vi "Display Hardware Devices.vi"(8 "error in (no error)":errorcluster, 9 "Hardware Type":string, 10 "Array of Hardware Device Names":string[](array[string]), 11 "Operator UI in":refnum<class "Measurement UI.lvclass">) -> (0 "error out":errorcluster, 3 "Operator UI out":refnum<class "Measurement UI.lvclass">)   [LabVIEW 2017, in "Measurement UI.lvlib" / "Measurement UI.lvclass"]
uses:
  Measurement UI.lvclass
  Measurement UI.lvclass/Measurement UI.ctl
  Read Multimeter.vi
  Accessors/Read Digitizer.vi
  Accessors/Read Function Generator.vi
  Accessors/Read Power Supply.vi
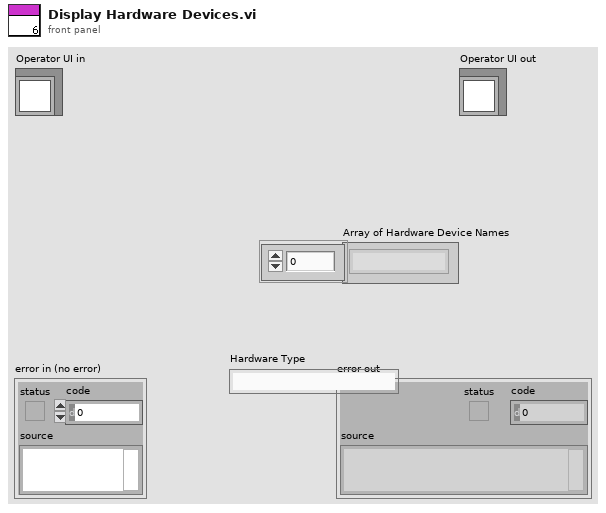
[diagram p1: front panel]
types:
  T1 = enum8{"Enabled", "Disabled", "Disabled and Grayed Out"}
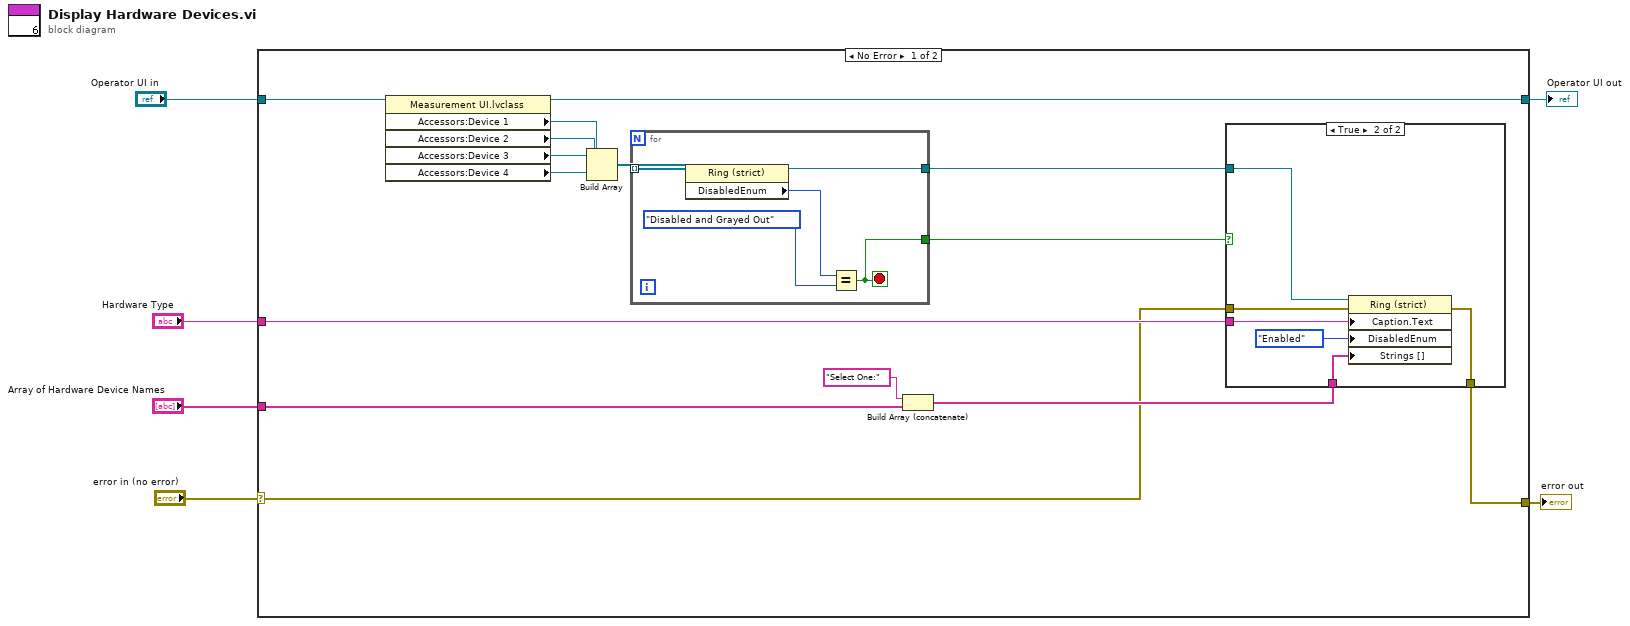
[diagram p0: block diagram]
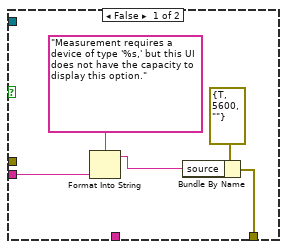
[diagram p2: hidden frame]
diagram:
  n1 = case shown="No Error" "error in (no error)" {
    selector: "error in (no error)" -> [w7 w39]
    tunnel: "Array of Hardware Device Names" -> [w21 _]
    tunnel: [w18 w39] -> w5
    tunnel: "Operator UI in" -> [w17 w38]
    tunnel: [w16 w38] -> w3
    tunnel: "Hardware Type" -> [w9 _]
    frame No Error {
      n2 = property class="Measurement UI.lvclass"(reference=w17) -> (reference out=w16:refnum<class "Measurement UI.lvclass">, "Accessors:Device 1"=w15:refnum<vi>, "Accessors:Device 2"=w14:refnum<vi>, "Accessors:Device 3"=w13:refnum<vi>, "Accessors:Device 4"=w12:refnum<vi>)  [unwired: 1 in, 1 out]
      n3 = Build Array(w15, w14, w13, w12) -> (w11:refnum<vi>[])
      n4 = for {
        tunnel: w11 -> [w26] mode=indexing
        tunnel: [w23] -> w10
        tunnel: [w22] -> w8
        stop <- w22 stop-if-true
        n5 = property class="Ring (strict)"(reference=w26) -> (reference out=w23:refnum<vi>, "DisabledEnum"=w25:T1)  [unwired: 1 in, 1 out]
        n6 = Equal?(x=w25, y=T1."Disabled and Grayed Out" ("Disabled")) -> (x = y?=w22:bool)
      }
      n7 = Build Array (concatenate)("Select One:" ("String"), w21) -> (w19:string[])
      n8 = case shown="True" w8 {
        tunnel: w19 -> [_ w37]
        tunnel: w10 -> [_ w36]
        tunnel: [w27 w34] -> w18
        tunnel: w9 -> [w28 w33]
        tunnel: w7 -> [_ w32]
        frame False {
          n9 = Format Into String(format string="Measurement requires a device of type '%s,' but this UI does not have the capacity to display this option.", w28) -> (resulting string=w30:string)  [unwired: 2 in, 1 out]
          n10 = Bundle By Name(cluster=errorcluster {"status"=TRUE, "code"=5600, "source"=""} ("error out"), "source"=w30) -> (w27:errorcluster)
        }
        frame True {
          n11 = property class="Ring (strict)"(reference=w36, error in=w32, "Caption.Text"=w33, "DisabledEnum"=T1."Enabled" ("Disabled"), "Strings []"=w37) -> (error out=w34:errorcluster)  [unwired: 1 out]
        }
      }
    }
    frame Error {
    }
  }
  "error out" <- w5
  "Operator UI out" <- w3
